vi "Error Converter (ErrCode or Status).vi"(8 "error in (no error)":errorcluster caption="Fehler (Eingang, kein Fehler)", 11 "error code":u32 caption="Fehlercode") -> (0 "error out":errorcluster caption="Fehler (Ausgang)")   [LabVIEW 2015, in "IRB.lvlib"]
uses:
  IRB.lvlib
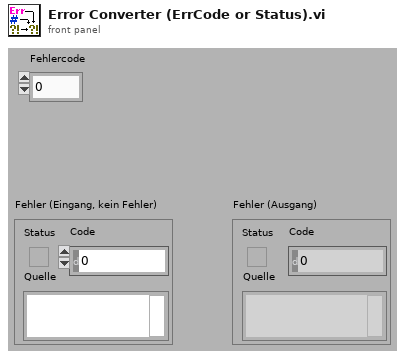
[diagram p1: front panel]
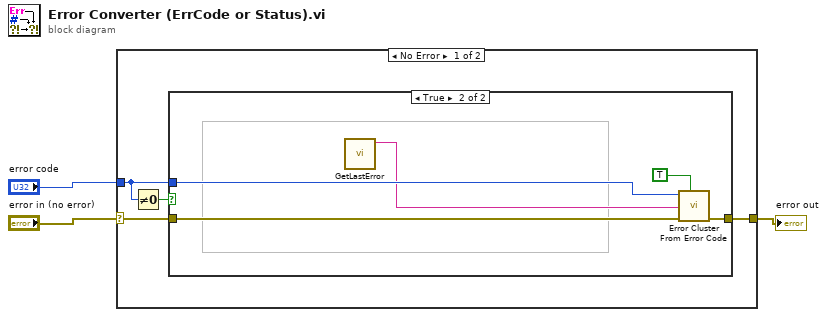
[diagram p0: block diagram]
diagram:
  n1 = case shown="No Error" "error in (no error)" {
    selector: "error in (no error)" -> [w6 w14]
    tunnel: [w4 w14] -> w2
    tunnel: "error code" -> [w5 _]
    frame No Error {
      n2 = Not Equal To 0?(x=w5) -> (x != 0?=w7:bool)
      n3 = case shown="True" w7 {
        tunnel: w6 -> [w8 w13]
        tunnel: w5 -> [_ w11]
        tunnel: [w8 w12] -> w4
        frame False {
        }
        frame True {
          n4 = call "GetLastError.vi"() -> ("function return"=w9:string)  [unwired: 11 in]
          n5 = call <vilib>:"Error Cluster From Error Code.vi"("show call chain? (False)"=TRUE, "error in (no error)"=w13, "error message (\"\")"=w9, "error code (0)"=w11) -> ("error out"=w12:errorcluster)  [unwired: 5 in]
        }
      }
    }
    frame Error {
    }
  }
  "error out" <- w2
